vi "Obtain ALL QUEUES.vi"(8 "error in (no error)":errorcluster) -> (0 "error out":errorcluster, 3 "Queues":T1)   [LabVIEW 2024]
uses:
  All Message Queues.ctl
  Message Cluster.ctl
  CTRLS/GLB_VAR.vi
  Message Queue.lvlib
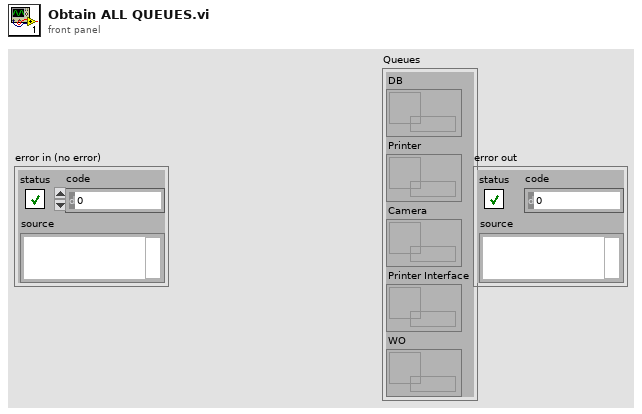
[diagram p1: front panel]
types:
  T1 = typedef "All Message Queues.ctl" = cluster{"DB":refnum<queue>, "Printer":refnum<queue>, "Camera":refnum<queue>, "Printer Interface":refnum<queue>, "WO":refnum<queue>}
  T2 = enum16{"Init SRL Buffer", "Insert SRL in Buffer", "Insert SRL Status", "Remove SRL from Buffer"}
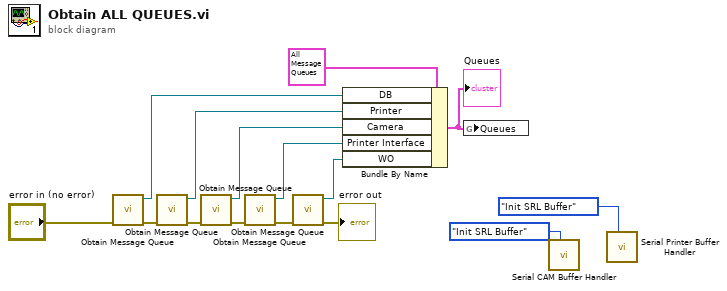
[diagram p0: block diagram]
diagram:
  n1 = call "Obtain Message Queue.vi"("error in (no error)"="error in (no error)") -> ("error out"=w11:errorcluster, "Message Queue"=w14:refnum<queue>)  [unwired: 9 in]
  n2 = call "Obtain Message Queue.vi"("error in (no error)"=w11) -> ("error out"=w10:errorcluster, "Message Queue"=w13:refnum<queue>)  [unwired: 9 in]
  n3 = call "Obtain Message Queue.vi"("error in (no error)"=w10) -> ("error out"=w6:errorcluster, "Message Queue"=w12:refnum<queue>)  [unwired: 9 in]
  n4 = call "Obtain Message Queue.vi"("error in (no error)"=w6) -> ("error out"=w5:errorcluster, "Message Queue"=w7:refnum<queue>)  [unwired: 9 in]
  n5 = call "Obtain Message Queue.vi"("error in (no error)"=w5) -> ("error out"=→"error out":errorcluster, "Message Queue"=w4:refnum<queue>)  [unwired: 9 in]
  n6 = Bundle By Name(cluster=T1 {"DB"=refnum, "Printer"=refnum, "Camera"=refnum, "Printer Interface"=refnum, "WO"=refnum} ("Message Queues"), "DB"=w14, "Printer"=w13, "Camera"=w12, "Printer Interface"=w7, "WO"=w4) -> (w9:T1)
  "Queues" <- w9
  n7 = global write "GLB_VAR.vi" "Queues"(w9) -> ()
  n8 = call "Serial CAM Buffer Handler.vi"("Serials buffer operations"=T2."Init SRL Buffer") -> ()  [unwired: 8 in, 3 out]
  n9 = call "Serial Printer Buffer Handler.vi"("Serials buffer operations"=T2."Init SRL Buffer") -> ()  [unwired: 9 in, 2 out]
